vi "Team Move.vi"(4 "MIA?[p]":bool[](array[boolean]), 6 "Confirmed?[p]":bool[](array[boolean]), 7 "Move Cnt":i32, 8 "error in (no error)":errorcluster, 9 "Player[p] in":T1[](array[typedef]), 10 "p[x][y]":i32[][](array[numeric]), 11 "BTeam in":refnum<class "BTeam.lvclass">) -> (0 "error out":errorcluster, 1 "Player[p] out":T1[](array[typedef]), 3 "BTeam out":refnum<class "BTeam.lvclass">)   [LabVIEW 2015, in "BTeam.lvclass"]
uses:
  BTeam.lvclass
  TeamEffort/private/Player Cluster.ctl
  Square/Square.lvclass
  TeamEffort/Team Move Input.ctl
  Type Defs/Action Enum.ctl
  TeamEffort/Team Move Output.ctl
  Type Defs/Direction Enum.ctl
  BTeam.lvclass/BTeam.ctl
  Type Defs/SB Type Defs.lvlib
  TeamEffort/TeamEffort.lvclass
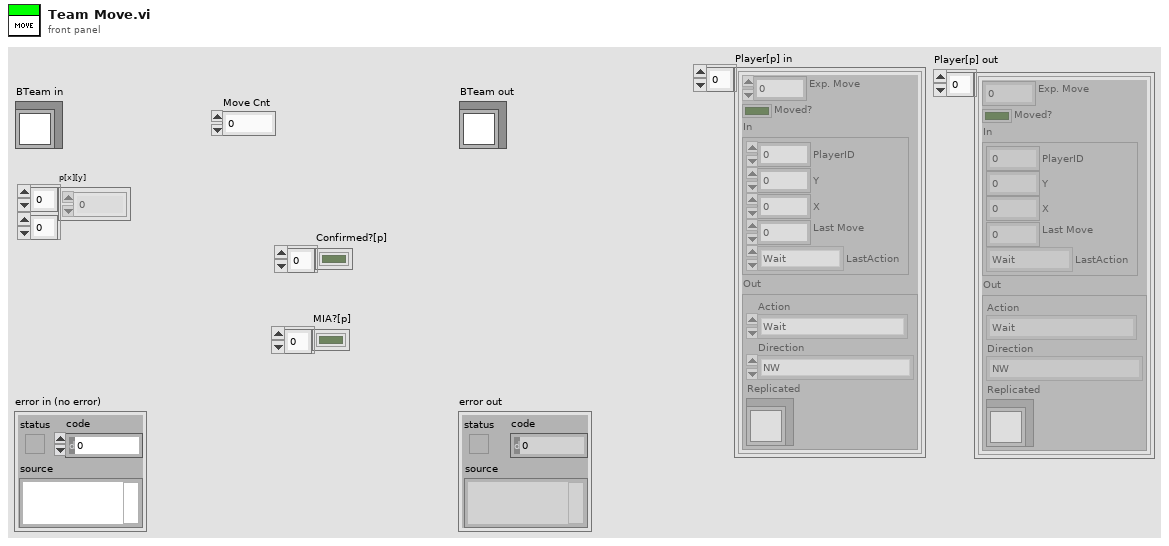
[diagram p1: front panel]
types:
  T1 = typedef "TeamEffort.lvclass/Player Cluster.ctl" = cluster{"Exp. Move":i32, "Moved?":bool, "In":T2, "Out":T4}
  T2 = typedef "TeamEffort.lvclass/Team Move Input.ctl" = cluster{"PlayerID":i32, "Y":i32, "X":i32, "Last Move":i32, "LastAction":T3}
  T3 = typedef "SB Type Defs.lvlib/Action Enum.ctl" = enum16{"Wait", "Move", "Attack", "Replicate"}
  T4 = typedef "TeamEffort.lvclass/Team Move Output.ctl" = cluster{"Action":T3, "Direction":T5, "Replicated":refnum<class "Square.lvclass">}
  T5 = typedef "SB Type Defs.lvlib/Direction Enum.ctl" = enum16{"NW", "N", "NE", "E", "SE", "S", "SW", "W"}
  T6 = typedef "BTeam.lvclass/Team Cluster.ctl" = cluster{"Mode":T7, "Y":i32, "X":i32, "Count":i32, "Dir":i32}
  T7 = typedef "BTeam.lvclass/Mode Enum.ctl" = enum16{"<Unknown>", "1", "2", "4", "8", "16", "Check", "Spawn"}
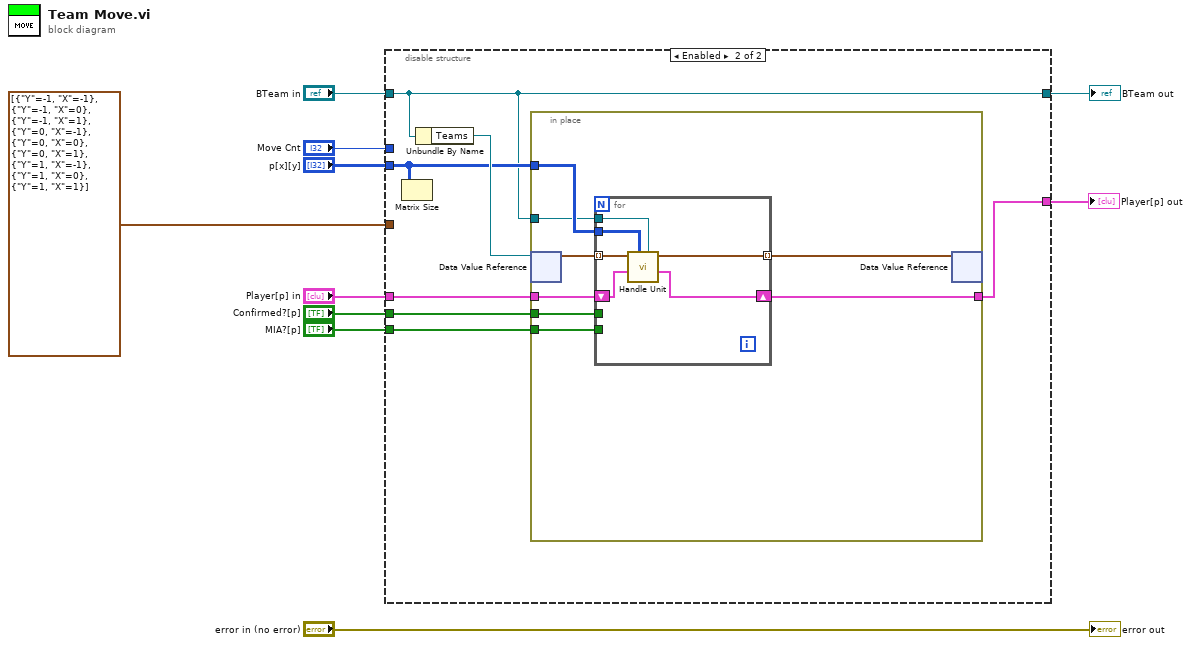
[diagram p0: block diagram]
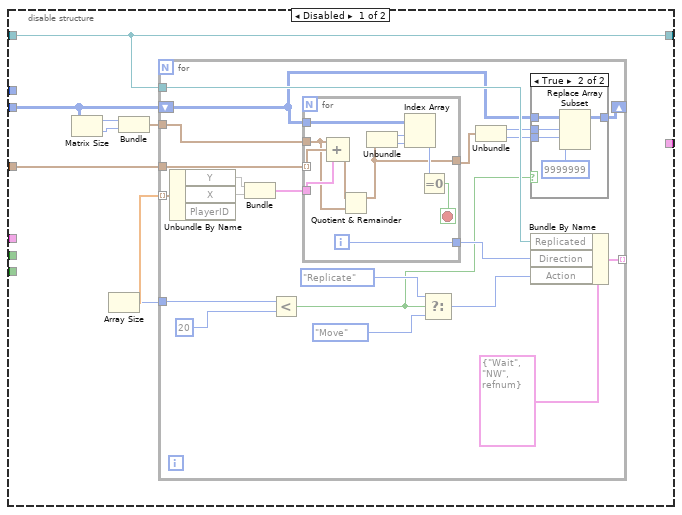
[diagram p2: hidden frame]
diagram:
  n1 = disable-structure shown="Enabled" {
    disable-tunnel: "BTeam in" -> [w11 w57]
    disable-tunnel: cluster{"Y":i32, "X":i32}[] [{"Y"=-1, "X"=-1}, {"Y"=-1, "X"=0}, {"Y"=-1, "X"=1}, {"Y"=0, "X"=-1}, {"Y"=0, "X"=0}, {"Y"=0, "X"=1}, {"Y"=1, "X"=-1}, {"Y"=1, "X"=0}, {"Y"=1, "X"=1}] -> [w16 _]
    disable-tunnel: [w11 w57] -> w7
    disable-tunnel: "Move Cnt" -> [_ _]
    disable-tunnel: "p[x][y]" -> [w15 w62]
    disable-tunnel: "Player[p] in" -> [_ w61]
    disable-tunnel: "Confirmed?[p]" -> [_ w60]
    disable-tunnel: "MIA?[p]" -> [_ w59]
    disable-tunnel: [_ w58] -> w1
    frame Disabled {
      n2 = Matrix Size(0:w15) -> (1:w14:i32, 2:w13:i32)
      n3 = Array Size() -> (array=w18:dbl[], size(s)=w17:i32)
      n4 = Bundle("number of columns"=w14, "matrix"=w13) -> (w12:cluster{"number of columns":i32, "matrix":i32})  [unwired: 1 in]
      n5 = for {
        tunnel: w18 -> [w39] mode=indexing
        tunnel: w17 -> [w38]
        tunnel: w11 -> [w35]
        tunnel: [w33] -> _ mode=indexing
        tunnel: w16 -> [w30]
        tunnel: w12 -> [w28]
        shift-right: [w22] -> _
        shift-left: w15 -> [w23]
        n6 = Unbundle By Name(w39) -> ("Y"=w26, "X"=w27)  [unwired: 1 out]
        n7 = Bundle("Y"=w26, "X"=w27) -> (w25:cluster{"Y":void, "X":void})  [unwired: 1 in]
        n8 = Less?(x=w38, y=20) -> (x < y?=w24:bool)
        n9 = for {
          tunnel: w23 -> [w56]
          tunnel: w30 -> [w52] mode=indexing
          tunnel: [w53] -> w29
          tunnel: w28 -> [w49]
          tunnel: w25 -> [w51]
          tunnel: [w46] -> w21
          i -> [w53]
          stop <- w54 stop-if-true
          n10 = Compound Arithmetic op=ADD(w49, w52, w51) -> (w50:cluster{i32, i32})
          n11 = Quotient & Remainder(x=w50, y=w49) -> (x-y*floor(x/y)=w46:cluster{i32, i32})  [unwired: 1 out]
          n12 = Unbundle(w46) -> (w48:i32, w47:i32)
          n13 = Index Array(array=w56, index (row)=w48, index (col)=w47) -> (element=w55:i32)
          n14 = Equal To 0?(x=w55) -> (x = 0?=w54:bool)
        }
        n15 = Select(t=Action_Enum."Replicate" ("Action"), s=w24, f=Action_Enum."Move" ("Action")) -> (s? t:f=w32:T3)
        n16 = Unbundle(w21) -> (w20:i32, w19:i32)
        n17 = case shown="True" w24 {
          tunnel: w23 -> [w40 w45]
          tunnel: [w40 w44] -> w22
          tunnel: w20 -> [_ w43]
          tunnel: w19 -> [_ w42]
          frame False {
          }
          frame True {
            n18 = Replace Array Subset(array=w45, new element=9999999 ("new element/subarray"), index (row)=w43, index (col)=w42) -> (w44:i32[][])
          }
        }
        n19 = Bundle By Name(cluster=T4 {"Action"=enum."Wait", "Direction"=enum."NW", "Replicated"=refnum} ("Cluster"), "Replicated"=w35, "Direction"=w29, "Action"=w32) -> (w33:T4)
      }
    }
    frame Enabled {
      n20 = Matrix Size(0:w62) -> ()  [unwired: 2 out]
      n21 = Unbundle By Name(w57) -> ("Teams"=w63:refnum<data-value>)
      n22 = in-place {
        in-place-border: w62 -> [w69]
        in-place-border: w61 -> [w68]
        in-place-border: w60 -> [w67]
        in-place-border: w59 -> [w66]
        in-place-border: [w65] -> w58
        in-place-border: w57 -> [w64]
        n23 = in-place-dvr #1(w63) -> (w71:T6[])  [unwired: 1 out]
        n24 = for {
          tunnel: w71 -> [w77] mode=indexing
          tunnel: [w76] -> w70 mode=indexing
          tunnel: w69 -> [w75]
          shift-right: [w73] -> w65
          shift-left: w68 -> [w74]
          tunnel: w67 -> [_]
          tunnel: w66 -> [_]
          tunnel: w64 -> [w72]
          n25 = call "Handle Unit.vi"("BTeam in"=w72, "p[x][y]"=w75, "Player[p] in"=w74, "Unit in"=w77) -> ("Player[p] out"=w73:T1[], "Unit out"=w76:T6)  [unwired: 6 in]
        }
        n26 = in-place-dvr #1(w70) -> ()  [unwired: 2 out]
      }
    }
  }
  "BTeam out" <- w7
  "Player[p] out" <- w1
  "error out" <- "error in (no error)"
